vi "SetFirstValLin.vi"(6 "PAYLOAD in":u32[](array[numeric])=[0, 0, 0, 0, 0, 0, 0, 0] format="%x", 8 "error in (no error)":errorcluster, 9 "DLC in":u32, 10 "IDENTIFIER in":u32 format="%x", 11 "gRPC ID in":T1) -> (0 "error out":errorcluster, 3 "gRPC ID out":T1)   [LabVIEW 2025, in "CAN-LIN Frame Generator.lvclass"]
uses:
  CAN-LIN Frame Generator.lvclass
  CAN-LIN Frame Generator.lvclass/CAN-LIN Frame Generator.ctl
  CAN-LIN Frame Generator UI/OOB gRPC Client/RPC Messages/hwval_GenericRequest.ctl
  CAN-LIN Frame Generator UI/OOB gRPC Client/OOB gRPC Client.lvlib
  <vilib>/gRPC/LabVIEW gRPC Library/Shared/grpcId.ctl
  <vilib>/gRPC/LabVIEW gRPC Library/grpc-lvsupport-release.lvlib
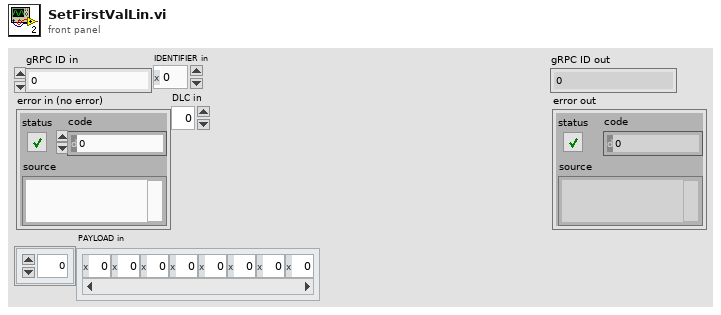
[diagram p1: front panel]
types:
  T1 = typedef "grpc-lvsupport-release.lvlib/grpcId.ctl" = u64
  T2 = typedef "OOB gRPC Client.lvlib/hwval_GenericRequest.ctl" = cluster{"Command":string, "Payload":u8[]}
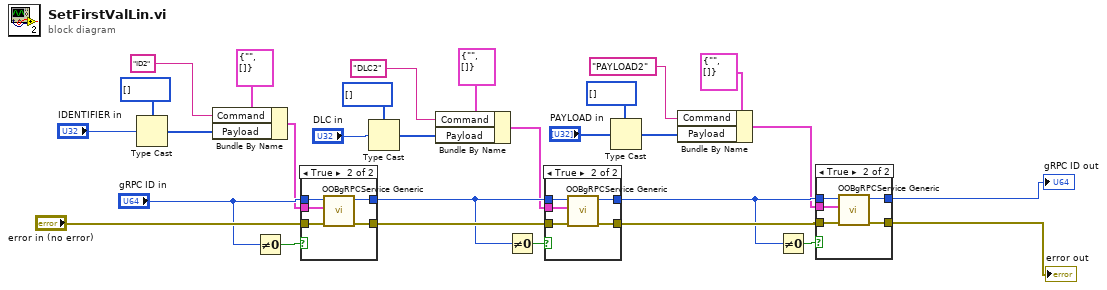
[diagram p0: block diagram]
diagram:
  n1 = Type Cast(type=u8[] [] ("Payload"), x="IDENTIFIER in") -> (*(type *) &x=w8:u8[])
  n2 = Bundle By Name(cluster=T2 {"Command"="", "Payload"=[]} ("hwval_GenericRequest"), "Command"="ID2", "Payload"=w8) -> (w17:T2)
  n3 = Not Equal To 0?(x="gRPC ID in") -> (x != 0?=w23:bool)
  n4 = case shown="True" w23 {
    tunnel: [w31 w33] -> w22
    tunnel: [w30 w32] -> w26
    tunnel: "gRPC ID in" -> [w31 w36]
    tunnel: "error in (no error)" -> [w30 w35]
    tunnel: w17 -> [_ w34]
    frame False {
    }
    frame True {
      n5 = call "OOBgRPCService Generic.vi"("error in"=w35, "Request Data"=w34, "gRPC ID"=w36) -> ("error out"=w32:errorcluster, "gRPC ID out"=w33:T1)  [unwired: 6 in, 1 out]
    }
  }
  n6 = Type Cast(type=u8[] [] ("Payload"), x="DLC in") -> (*(type *) &x=w6:u8[])
  n7 = Bundle By Name(cluster=T2 {"Command"="", "Payload"=[]} ("hwval_GenericRequest"), "Command"="DLC2", "Payload"=w6) -> (w13:T2)
  n8 = Not Equal To 0?(x=w22) -> (x != 0?=w21:bool)
  n9 = case shown="True" w21 {
    tunnel: [w38 w40] -> w19
    tunnel: [w37 w39] -> w27
    tunnel: w22 -> [w38 w43]
    tunnel: w26 -> [w37 w42]
    tunnel: w13 -> [_ w41]
    frame False {
    }
    frame True {
      n10 = call "OOBgRPCService Generic.vi"("error in"=w42, "Request Data"=w41, "gRPC ID"=w43) -> ("error out"=w39:errorcluster, "gRPC ID out"=w40:T1)  [unwired: 6 in, 1 out]
    }
  }
  n11 = Type Cast(type=u8[] [] ("Payload"), x="PAYLOAD in") -> (*(type *) &x=w4:u8[])
  n12 = Bundle By Name(cluster=T2 {"Command"="", "Payload"=[]} ("hwval_GenericRequest"), "Command"="PAYLOAD2", "Payload"=w4) -> (w14:T2)
  n13 = Not Equal To 0?(x=w19) -> (x != 0?=w20:bool)
  n14 = case shown="True" w20 {
    tunnel: [w45 w47] -> w29
    tunnel: [w44 w46] -> w28
    tunnel: w19 -> [w45 w50]
    tunnel: w27 -> [w44 w49]
    tunnel: w14 -> [_ w48]
    frame False {
    }
    frame True {
      n15 = call "OOBgRPCService Generic.vi"("error in"=w49, "Request Data"=w48, "gRPC ID"=w50) -> ("error out"=w46:errorcluster, "gRPC ID out"=w47:T1)  [unwired: 6 in, 1 out]
    }
  }
  "gRPC ID out" <- w29
  "error out" <- w28
